vi "Cluster Experiment.vi"() -> ()   [LabVIEW 2014]
panel:
  out "Small Cluster":cluster{"Boolean 1":bool, "Slide Value":dbl}
  out "Modified Cluster":T1 {"Slide" scale=0.0..10.0}
  in  "Cluster":T1 {"Slide" scale=0.0..10.0}
  out "Boolean 2":bool
  out "Numeric":dbl
  in  "stop":bool
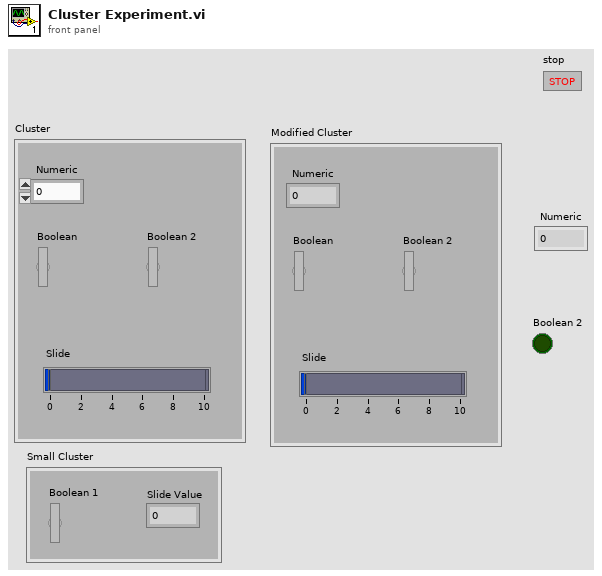
[diagram p1: front panel]
types:
  T1 = cluster{"Numeric":dbl, "Boolean":bool, "Boolean 2":bool, "Slide":dbl}
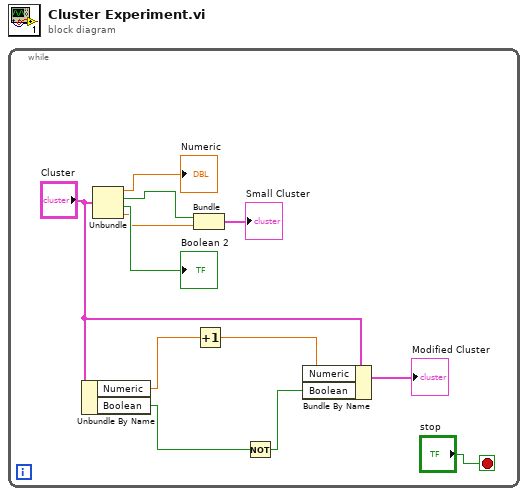
[diagram p0: block diagram]
diagram:
  n1 = while {
    stop <- "stop" stop-if-true
    n2 = Unbundle By Name("Cluster") -> ("Numeric"=w5:dbl, "Boolean"=w6:bool)
    n3 = Unbundle("Cluster") -> ("Numeric"=→"Numeric":dbl, "Boolean"=w9:bool, "Boolean 2"=→"Boolean 2":bool, "Slide"=w7:dbl)
    n4 = Bundle("Boolean"=w9, "Slide"=w7) -> (→"Small Cluster":cluster{"Boolean":bool, "Slide":dbl})  [unwired: 1 in]
    n5 = Increment(x=w5) -> (x+1=w3:dbl)
    n6 = Not(x=w6) -> (.not. x?=w4:bool)
    n7 = Bundle By Name(cluster="Cluster", "Numeric"=w3, "Boolean"=w4) -> (→"Modified Cluster":T1)
  }
